vi "Get Base Command.vi"(8 "error in (no error)":errorcluster, 11 "Instrument in":refnum<class "Instrument.lvclass">) -> (0 "error out":errorcluster, 2 "Base Command":string, 3 "Instrument out":refnum<class "Instrument.lvclass">)   [LabVIEW 2023, in "HAF.lvlib" / "Instrument.lvclass"]
doc: "Returns the base command whch is used to build up the overall command string – parameters will be added to this as necessary.  The framework will add the line terminator \\n.\n\nSubclasses MUST override this member and must not add a line terminator on the end of the command; on this class an error is returned."
uses:
  Instrument.lvclass
  Instrument.lvclass/Instrument.ctl
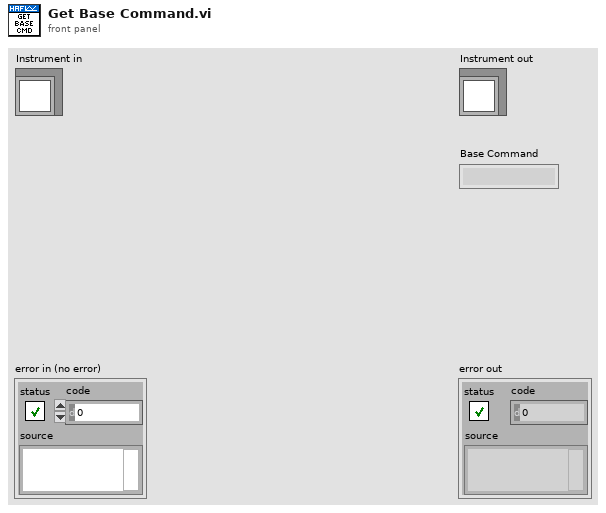
[diagram p1: front panel]
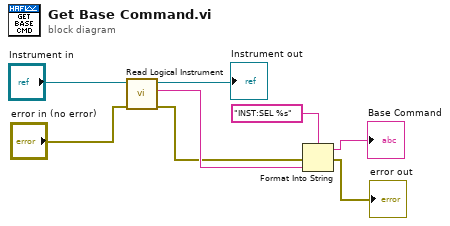
[diagram p0: block diagram]
diagram:
  n1 = call-dynamic "Read Logical Instrument.vi"("error in (no error)"="error in (no error)", "Instrument in"="Instrument in") -> ("error out"=w4:errorcluster, "Logical Instrument"=w5:string, "Instrument out"=→"Instrument out":refnum<class "Instrument.lvclass">)  [unwired: 7 in]
  n2 = Format Into String(format string="INST:SEL %s", error in=w4, w5) -> (resulting string=→"Base Command":string, error out=→"error out":errorcluster)  [unwired: 1 in]
